vi "Configure Curr Trigger.vi"(8 "error in (no error)":errorcluster, 10 "Curr Trigger(0)":dbl=45.0 min=0.0 max=300.0, 11 "VISA resource name":refnum<visa-resource-name>) -> (0 "error out":errorcluster, 3 "VISA resource name out":refnum<visa-resource-name>)   [LabVIEW 2020, in "IT6500.lvlib"]
doc: "The command is used to set a current value that is waiting to be triggered.This value is stored until a trigger letter is received\nThe power supply is then exported by the current value.Sending the <b>CURRent</b> command does not affect the value set by this command.\nThe value that was set before the query command is sent back."
uses:
  IT6500.lvlib
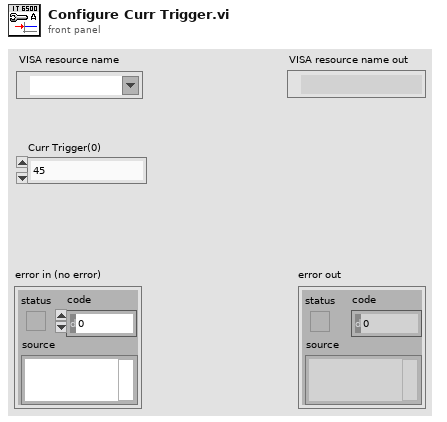
[diagram p1: front panel]
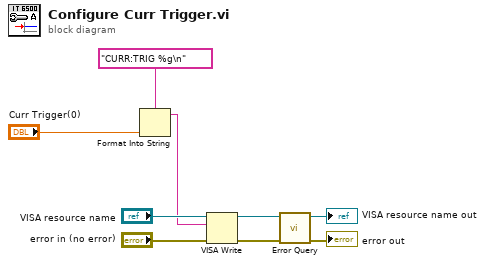
[diagram p0: block diagram]
diagram:
  n1 = Format Into String(format string="CURR:TRIG %g\n", "Curr Trigger(0)") -> (resulting string=w3:string)  [unwired: 2 in, 1 out]
  n2 = VISA Write(VISA resource name="VISA resource name", write buffer=w3, error in (no error)="error in (no error)") -> (VISA resource name out=w6:refnum<visa-resource-name>, error out=w7:errorcluster)  [unwired: 1 out]
  n3 = call "Error Query.vi"("error in (no error)"=w7, "VISA resource name"=w6) -> ("error out"=→"error out":errorcluster, "VISA resource name out"=→"VISA resource name out":refnum<visa-resource-name>)  [unwired: 6 in, 2 out]
